vi "Handle Errors.vi"(8 "error in (no error)":errorcluster, 10 "Error Message Data":T1, 11 "Error Handler In":refnum<class "Error Handler.lvclass">) -> (0 "error out":errorcluster, 3 "Error Handler Out":refnum<class "Error Handler.lvclass">)   [LabVIEW 2020, in "Error Handler.lvclass"]
doc: "Critical errors are sent to registered processes where they should be handled by the error case. Fatal errors stops the regsitered processes. All errors not in the severity map are logged to file."
uses:
  Error Handler.lvclass
  Public/TypeDefs/Error Message Data.ctl
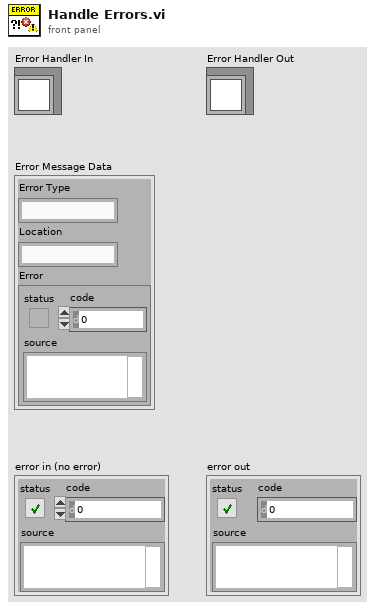
[diagram p1: front panel]
types:
  T1 = typedef "Error Handler.lvclass/Error Message Data.ctl" = cluster{"Error Type":string, "Location":string, "Error":errorcluster}
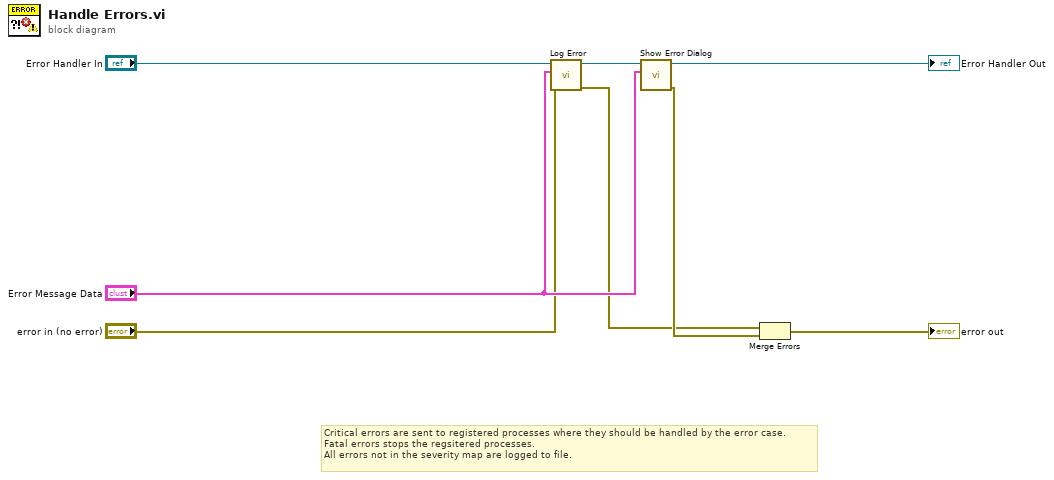
[diagram p0: block diagram]
diagram:
  # "Critical errors are sent to registered processes where they should be handled by the error case.\nFatal errors stops the regsitered processes.\nAll errors not in the severity map are logged to file."
  n1 = call "Log Error.vi"("error in (no error)"="error in (no error)", "Error Message Data"="Error Message Data", "Error Handler In"="Error Handler In") -> ("error out"=w2:errorcluster, "Error Handler Out"=w4:refnum<class "Error Handler.lvclass">)  [unwired: 7 in]
  n2 = call "Show Error Dialog.vi"("Error Message Data"="Error Message Data", "Error Handler In"=w4) -> ("error out"=w3:errorcluster, "Error Handler Out"=→"Error Handler Out":refnum<class "Error Handler.lvclass">)  [unwired: 8 in]
  n3 = Merge Errors(w2, w3) -> (→"error out":errorcluster)
